vi "Length_9.vi"() -> ()   [LabVIEW 2020]
uses:
  Support/Controls/Cmd_Mouse Popup.ctl
  Support/Controls/Clst_Initialize Input.ctl
  Support/Controls/Cmd_Var Data IO.ctl
  Variables/Global_Cal Info.vi
panel:
  out "Spec 2":string[][](table) caption="Spec"
  out "Measured 2":string[][](table) caption="참고데이터"
  in  "체눈 수":string="10"
  in  "단위":string(combo)
  in  "선재 지름":string
  in  "체눈 크기":string
  in  "Spec 변경":bool
  in  "Random":bool
  out "Spec":string[][](table) caption="Spec Default"
  out "제목":string
  out "에러 출력":errorcluster
  out "Condition":string[][](table) caption="2. 직선성 시험"
  in  "Measured":string[][](table) caption="측정결과"
  out "Load?":bool
  # "※ 참고데이터는 기준기 보정값 적용하지 않은 체눈크기 계산 후 값임."
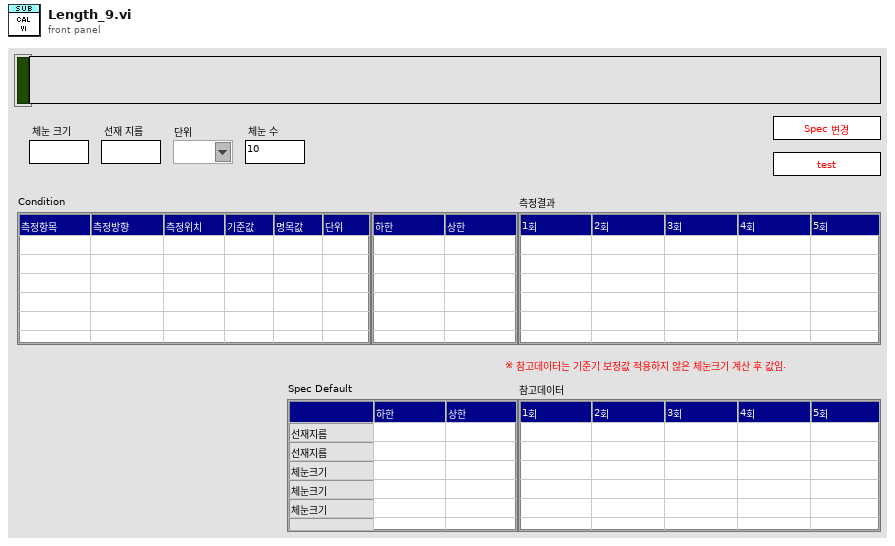
[diagram p1: front panel]
types:
  T1 = typedef "Cmd_Mouse Popup.ctl" = enum16{"활성화", "메뉴선택"}
  T2 = cluster{"Shift":bool, "Ctrl":bool, "Alt":bool, "Cmd":bool, "Opt":bool}
  T3 = typedef "Clst_Initialize Input.ctl" = cluster{"Initialize 1":cluster{"Condition":refnum<vi>[], "Spec":refnum<vi>[], "Measured":refnum<vi>[], "Resolution":refnum<vi>[], "Func_ext":string, "제목":refnum<vi>, "Measured_ADJ":refnum<vi>[]}, "Initialize 2":cluster{"문자열":refnum<vi>[], "콤보박스":refnum<vi>[], "링":refnum<vi>[], "열거형":refnum<vi>[], "테이블":refnum<vi>[], "여러열":refnum<vi>[], "디지털(DBL)":refnum<vi>[], "3D string":refnum<vi>[], "ctrl":refnum<vi>[], "boolean":refnum<vi>[]}}
  T4 = typedef "Cmd_Var Data IO.ctl" = enum16{"Condition", "Condition Default", "Condition_Temp", "Resolution", "Resolution Default", "Resolution Old", "Spec", "Spec Default", "Spec Old", "Spec Temp", "Result", "Result2", "Result3", "Result_Temp", "Result_ADJ", "Result_ADJ2", "STD1", "STD2", "STD3", "STD4", "STD5", "STD Temp", "CMC", "CMC Default"}
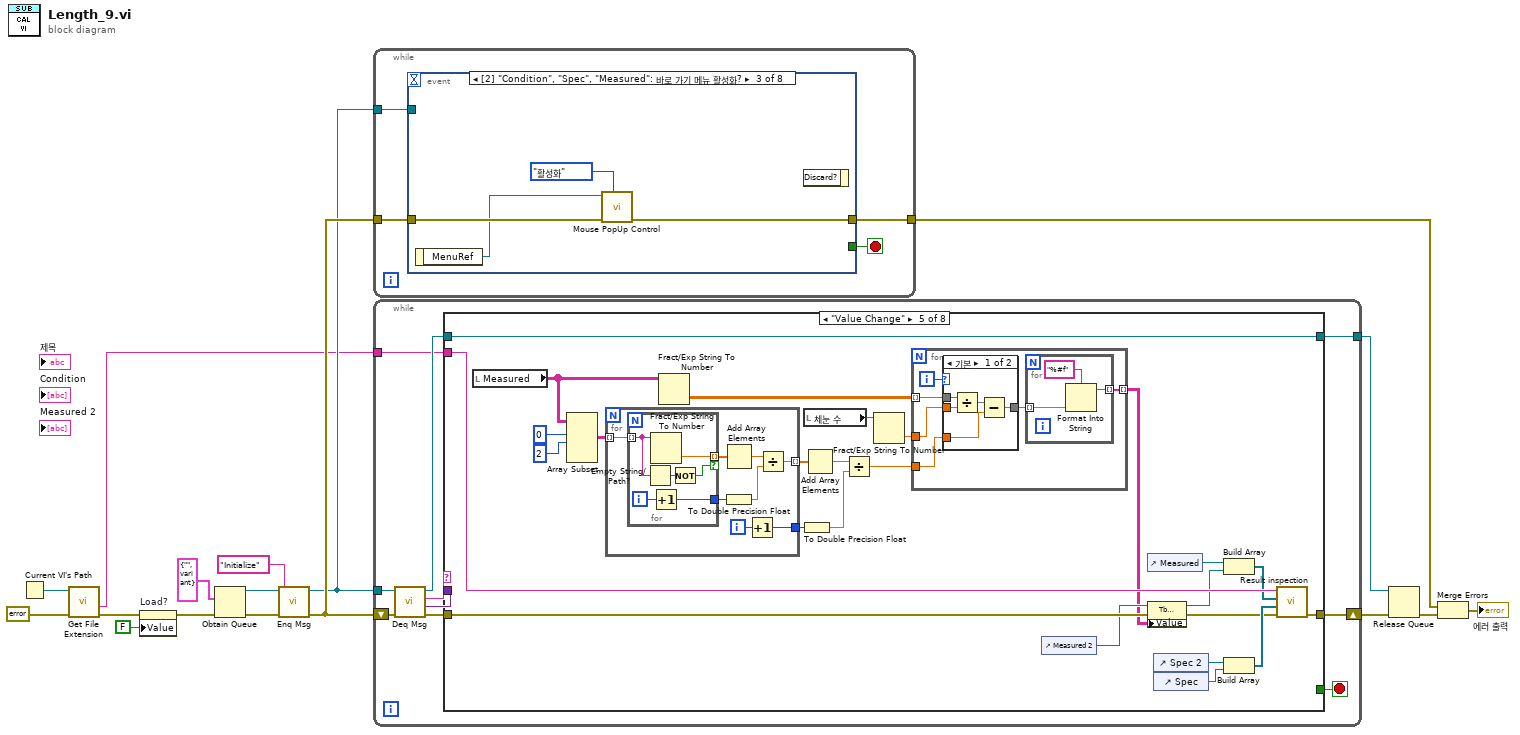
[diagram p0: block diagram]
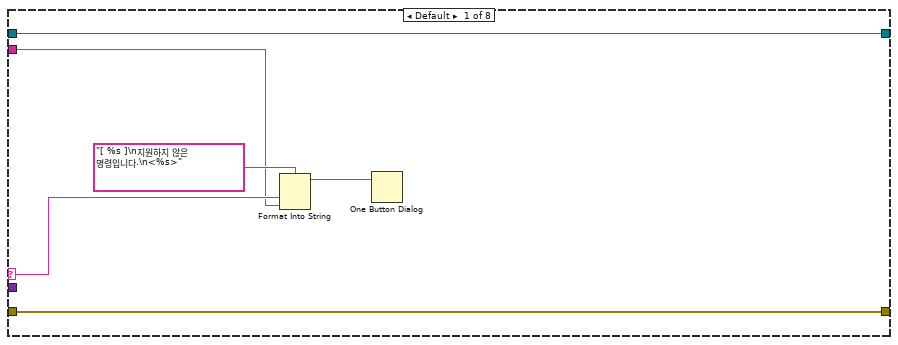
[diagram p2: hidden frame]
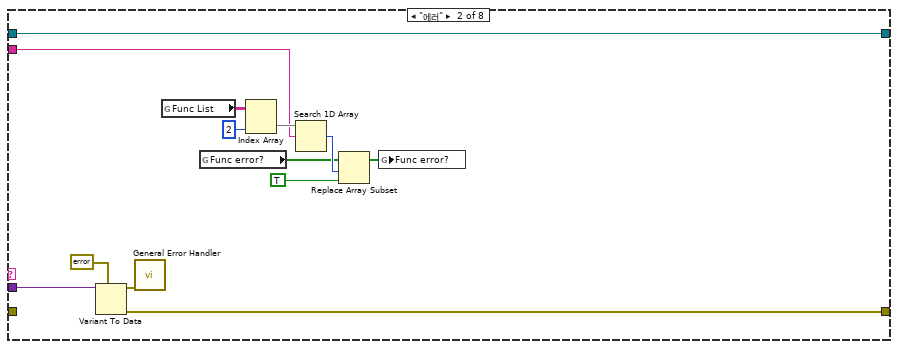
[diagram p3: hidden frame]
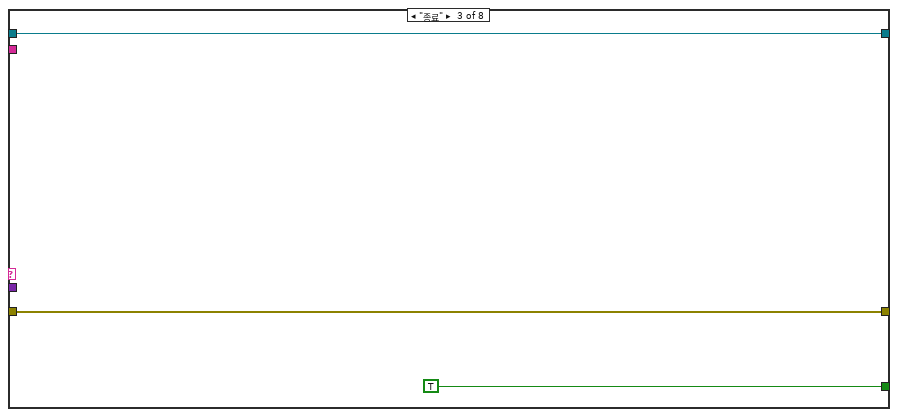
[diagram p4: hidden frame]
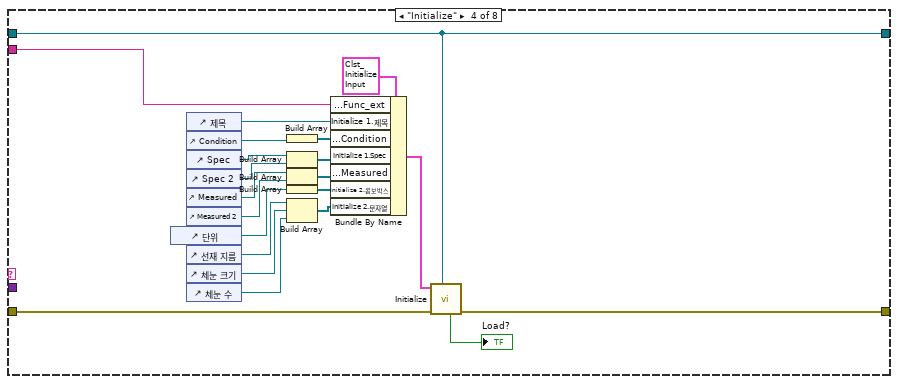
[diagram p5: hidden frame]
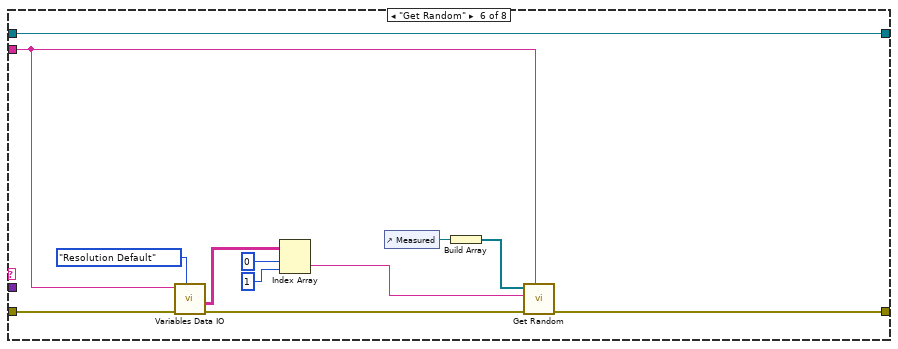
[diagram p7: hidden frame]
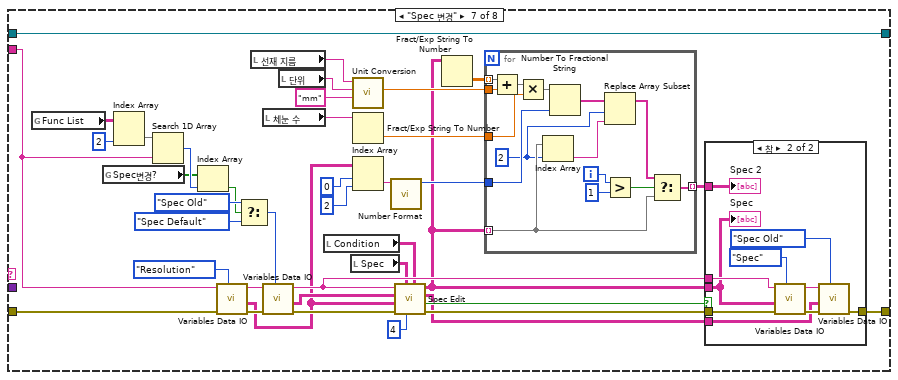
[diagram p8: hidden frame]
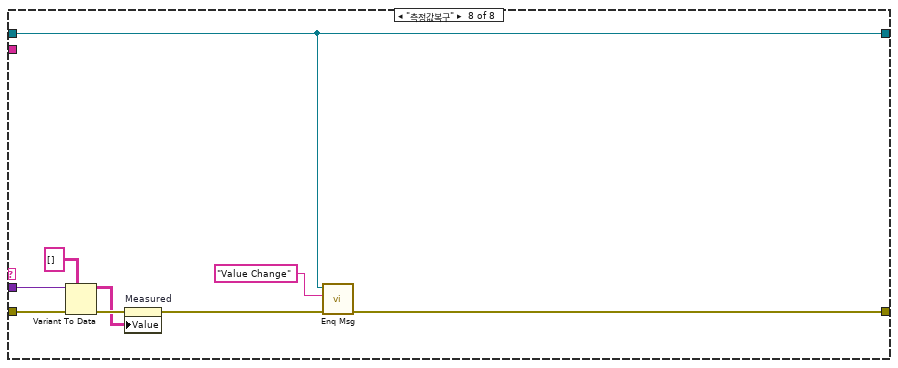
[diagram p10: hidden frame]
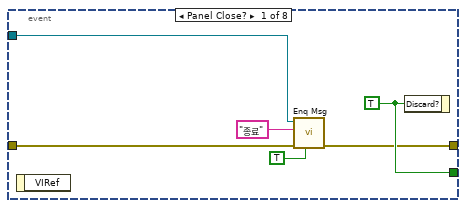
[diagram p11: hidden frame]
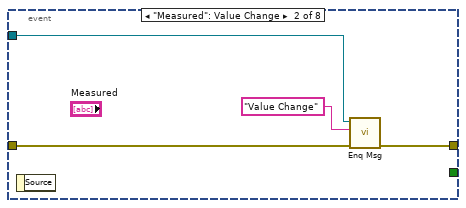
[diagram p12: hidden frame]
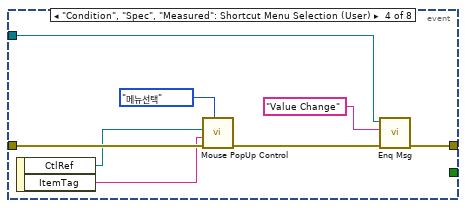
[diagram p13: hidden frame]
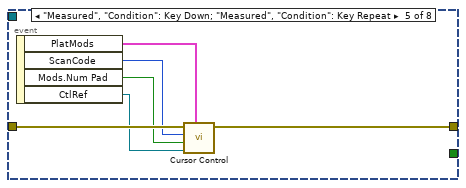
[diagram p14: hidden frame]
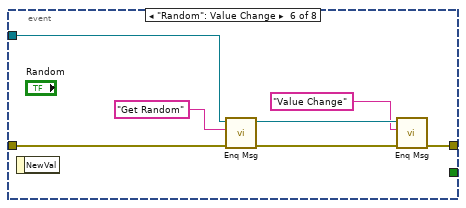
[diagram p15: hidden frame]
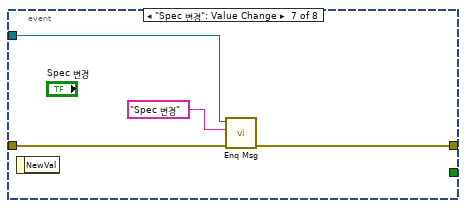
[diagram p16: hidden frame]
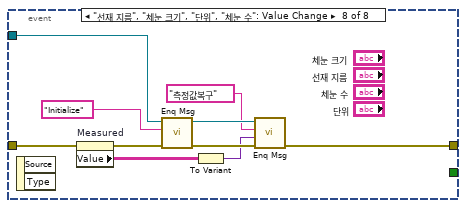
[diagram p17: hidden frame]
diagram:
  n1 = Current VI's Path() -> (path=w5:path)
  n2 = call <vilib>:"Get File Extension.vi"("error in (no error)"=errorcluster {"status"=FALSE, "code"=0, "source"=""} ("에러 상수"), "file"=w5) -> ("error out"=w3:errorcluster, "filename without extension"=w4:string)  [unwired: 5 in, 3 out]
  n3 = property on="Load?" class="Bool (엄격한)"(error in=w3, "Value"=FALSE ("Load?")) -> (error out=w2:errorcluster)  [unwired: 1 in, 1 out]
  n4 = Obtain Queue(element data type=cluster{"메세지":string, "값":variant} {"메세지"="", "값"=variant} ("Message Cluster"), error in (no error)=w2) -> (queue out=w14:refnum<queue>, error out=w16:errorcluster)  [unwired: 3 in, 1 out]
  n5 = call "Enq Msg.vi"("에러 입력(에러 없음)"=w16, "메세지"="Initialize", "큐 입력"=w14) -> ("에러 출력"=w15:errorcluster, "큐 출력"=w12:refnum<queue>)  [unwired: 7 in]
  n6 = while {
    tunnel: w15 -> [w19]
    tunnel: w12 -> [w20]
    tunnel: [w18] -> w9
    stop <- w21 stop-if-true
    n7 = event shown="[2] \"Condition\", \"Spec\", \"Measured\": 바로 가기 메뉴 활성화?" {
      selector: _ -> [_ _ _ _ _ _ _ _]
      dyn-events: _ -> [_ _ _ _ _ _ _ _]
      timeout: _ -> [_ _ _ _ _ _ _ _]
      tunnel: [w27 _ _ _ _ _ _ _] -> w21
      tunnel: w20 -> [w25 w31 _ w36 _ w54 w58 w69]
      tunnel: w19 -> [w26 w29 w35 w43 w49 w55 w59 w68]
      tunnel: [w23 w30 w34 w37 w48 w50 w57 w65] -> w18
      event Panel Close? {
        w27 = TRUE ("버림?")
        n8 = event-data() -> ()  [unwired: 1 in, 1 out]
        n9 = call "Enq Msg.vi"("우선순위 메시지?"=TRUE, "에러 입력(에러 없음)"=w26, "메세지"="종료", "큐 입력"=w25) -> ("에러 출력"=w23:errorcluster)  [unwired: 6 in, 1 out]
        n10 = event-data("Discard?"=w27) -> ()  [unwired: 1 in, 1 out]
      }
      event "Measured": Value Change {
        n11 = event-data() -> ()  [unwired: 1 in, 1 out]
        n12 = call "Enq Msg.vi"("에러 입력(에러 없음)"=w29, "메세지"="Value Change", "큐 입력"=w31) -> ("에러 출력"=w30:errorcluster)  [unwired: 7 in, 1 out]
      }
      event "Condition", "Spec", "Measured": Shortcut Menu Activation? {
        n13 = event-data() -> ("MenuRef"=w33:refnum<k9>)  [unwired: 1 in]
        n14 = call "Mouse PopUp Control.vi"("type"=Cmd_Mouse_Popup."활성화", "error in"=w35, "메뉴 참조"=w33) -> ("error out"=w34:errorcluster)  [unwired: 8 in]
        n15 = event-data() -> ()  [unwired: 2 in, 1 out]
      }
      event "Condition", "Spec", "Measured": Shortcut Menu Selection (User) {
        n16 = event-data() -> ("CtlRef"=w41:refnum<vi>, "ItemTag"=w40:string)  [unwired: 1 in]
        n17 = call "Mouse PopUp Control.vi"("type"=Cmd_Mouse_Popup."메뉴선택", "error in"=w43, "아이템 태그"=w40, "Tbl 참조 번호"=w41) -> ("error out"=w38:errorcluster)  [unwired: 7 in]
        n18 = call "Enq Msg.vi"("에러 입력(에러 없음)"=w38, "메세지"="Value Change", "큐 입력"=w36) -> ("에러 출력"=w37:errorcluster)  [unwired: 7 in, 1 out]
      }
      event "Measured", "Condition": Key Down; "Measured", "Condition": Key Repeat {
        n19 = event-data() -> ("PlatMods"=w44:T2, "ScanCode"=w47:i16, "Mods.Num Pad"=w46:bool, "CtlRef"=w45:refnum<vi>)  [unwired: 1 in]
        n20 = call "Cursor Control.vi"("플랫폼 조합키"=w44, "참조"=w45, "Num Pad"=w46, "ScanCode"=w47, "error in"=w49) -> ("error out"=w48:errorcluster)  [unwired: 5 in, 1 out]
      }
      event "Random": Value Change {
        n21 = event-data() -> ()  [unwired: 1 in, 1 out]
        n22 = call "Enq Msg.vi"("에러 입력(에러 없음)"=w55, "메세지"="Get Random", "큐 입력"=w54) -> ("에러 출력"=w53:errorcluster, "큐 출력"=w52:refnum<queue>)  [unwired: 7 in]
        n23 = call "Enq Msg.vi"("에러 입력(에러 없음)"=w53, "메세지"="Value Change", "큐 입력"=w52) -> ("에러 출력"=w50:errorcluster)  [unwired: 7 in, 1 out]
      }
      event "Spec 변경": Value Change {
        n24 = event-data() -> ()  [unwired: 1 in, 1 out]
        n25 = call "Enq Msg.vi"("에러 입력(에러 없음)"=w59, "메세지"="Spec 변경", "큐 입력"=w58) -> ("에러 출력"=w57:errorcluster)  [unwired: 7 in, 1 out]
      }
      event "선재 지름", "체눈 크기", "단위", "체눈 수": Value Change {
        n26 = event-data() -> ()  [unwired: 1 in, 2 out]
        n27 = property on="Measured" class="Tbl (엄격한)"(error in=w68) -> (error out=w67:errorcluster, "Value"=w61:string[][])  [unwired: 1 in, 1 out]
        n28 = call "Enq Msg.vi"("에러 입력(에러 없음)"=w67, "메세지"="Initialize", "큐 입력"=w69) -> ("에러 출력"=w66:errorcluster, "큐 출력"=w64:refnum<queue>)  [unwired: 7 in]
        n29 = To Variant(anything=w61) -> (Variant=w62:variant)
        n30 = call "Enq Msg.vi"("에러 입력(에러 없음)"=w66, "값"=w62, "메세지"="측정값복구", "큐 입력"=w64) -> ("에러 출력"=w65:errorcluster)  [unwired: 6 in, 1 out]
      }
    }
  }
  n31 = while {
    shift-right: [w80] -> w11
    shift-left: w15 -> [w79]
    tunnel: w12 -> [w77]
    tunnel: [w72] -> w10
    tunnel: w4 -> [w71]
    stop <- w73 stop-if-true
    n32 = call "Deq Msg.vi"("에러 입력(에러 없음)"=w79, "큐 입력"=w77) -> ("에러 출력"=w78:errorcluster, "값"=w74:variant, "메세지"=w76:string, "큐 출력"=w75:refnum<queue>)  [unwired: 6 in]
    n33 = case shown="\"Value Change\"" w76 {
      selector: w76 -> [w82 _ _ _ _ _ _ _]
      tunnel: w78 -> [w86 _ w102 w110 w137 w186 w209 w264]
      tunnel: [w86 w96 w102 w106 w148 w187 w226 w257] -> w80
      tunnel: w75 -> [w85 w95 w100 w114 w149 w190 w229 w256]
      tunnel: w74 -> [_ w97 _ _ _ _ _ w263]
      tunnel: [_ _ TRUE ("버림?") _ _ _ _ _] -> w73
      tunnel: [w85 w95 w100 w114 w149 w190 w229 w256] -> w72
      tunnel: w71 -> [w81 w87 _ w107 w147 w183 w207 _]
      frame Default {
        n34 = Format Into String(format string="[ %s ]\n지원하지 않은 명령입니다.\n<%s>" ("메시지"), w82, w81) -> (resulting string=w83:string)  [unwired: 2 in, 1 out]
        n35 = One Button Dialog(message=w83) -> ()  [unwired: 1 in, 1 out]
      }
      frame "에러" {
        n36 = Variant To Data(type=errorcluster {"status"=FALSE, "code"=0, "source"=""} ("에러 출력"), Variant=w97) -> (data=w99:errorcluster, error out=w96:errorcluster)  [unwired: 1 in]
        n37 = call <vilib>:"General Error Handler.vi"("error in (no error)"=w99) -> ()  [unwired: 10 in, 5 out]
        n38 = global read "Global_Cal Info.vi" "Func List"() -> (w89:string[][])
        n39 = global read "Global_Cal Info.vi" "Func error?"() -> (w92:bool[])
        n40 = Index Array(array=w89, index (col)=2 ("비활성화된 인덱스 (열)")) -> (element=w90:string[])  [unwired: 1 in]
        n41 = Search 1D Array(1D array=w90, element=w87) -> (index of element=w93:i32)  [unwired: 1 in]
        n42 = Replace Array Subset(array=w92, new element=TRUE ("새 원소/부분배열"), index=w93) -> (w94:bool[])
        n43 = global write "Global_Cal Info.vi" "Func error?"(w94) -> ()
      }
      frame "종료" {
      }
      frame "Initialize" {
        n44 = control-ref of="단위"() -> (w109:refnum<vi>)
        n45 = control-ref of="제목"() -> (w117:refnum<vi>)
        n46 = control-ref of="Condition"() -> (w122:refnum<vi>)
        n47 = control-ref of="Spec"() -> (w116:refnum<vi>)
        n48 = control-ref of="Spec 2"() -> (w105:refnum<vi>)
        n49 = control-ref of="Measured"() -> (w119:refnum<vi>)
        n50 = control-ref of="Measured 2"() -> (w104:refnum<vi>)
        n51 = control-ref of="선재 지름"() -> (w111:refnum<vi>)
        n52 = control-ref of="체눈 크기"() -> (w112:refnum<vi>)
        n53 = control-ref of="체눈 수"() -> (w108:refnum<vi>)
        n54 = Build Array(w122) -> (w121:refnum<vi>[])
        n55 = Build Array(w116, w105) -> (w115:refnum<vi>[])
        n56 = Build Array(w119, w104) -> (w120:refnum<vi>[])
        n57 = Build Array(w109) -> (w118:refnum<vi>[])
        n58 = Build Array(w111, w112, w108) -> (w113:refnum<vi>[])
        n59 = Bundle By Name(cluster=T3 {"Initialize 1"={"Condition"=[], "Spec"=[], "Measured"=[], "Resolution"=[], "Func_ext"="", "제목"=refnum, "Measured_ADJ"=[]}, "Initialize 2"={"문자열"=[], "콤보박스"=[], "링"=[], "열거형"=[], "테이블"=[], "여러열"=[], "디지털(DBL)"=[], "3D string"=[], "ctrl"=[], "boolean"=[]}} ("입력 클러스터"), "Initialize 1.Func_ext"=w107, "Initialize 1.제목"=w117, "Initialize 1.Condition"=w121, "Initialize 1.Spec"=w115, "Initialize 1.Measured"=w120, "Initialize 2.콤보박스"=w118, "Initialize 2.문자열"=w113) -> (w123:T3)
        n60 = call "Initialize.vi"("큐 입력"=w114, "error in"=w110, "입력 클러스터"=w123) -> ("error out"=w106:errorcluster, "Load?"=→"Load?":bool)  [unwired: 5 in, 2 out]
      }
      frame "Value Change" {
        n61 = local read "Measured"() -> (w130:string[][])
        n62 = Array Subset(array=w130, index (row)=0 ("인덱스"), length (row)=2 ("길이")) -> (w138:string[][])  [unwired: 2 in]
        n63 = for {
          tunnel: w138 -> [w155] mode=indexing
          tunnel: [w156] -> w129 mode=indexing
          tunnel: [w150] -> w128
          i -> [w151]
          n64 = for {
            tunnel: w155 -> [w163] mode=indexing
            tunnel: [w162] -> w154 mode=indexing if=w160
            tunnel: [w158] -> w153
            i -> [w159]
            n65 = Empty String/Path?(string/path=w163) -> (empty?=w161:bool)
            n66 = Fract/Exp String To Number(string=w163) -> (number=w162:dbl)  [unwired: 3 in, 1 out]
            n67 = Increment(x=w159) -> (x+1=w158:i32)
            n68 = Not(x=w161) -> (.not. x?=w160:bool)
          }
          n69 = Add Array Elements(numeric array=w154) -> (sum=w157:dbl)
          n70 = To Double Precision Float(number=w153) -> (double precision float=w152:dbl)
          n71 = Increment(x=w151) -> (x+1=w150:i32)
          n72 = Divide(x=w157, y=w152) -> (x/y=w156:dbl)
        }
        n73 = Fract/Exp String To Number(string=w130) -> (number=w141:dbl[][])  [unwired: 3 in, 1 out]
        n74 = To Double Precision Float(number=w128) -> (double precision float=w126:dbl)
        n75 = local read "체눈 수"() -> (w132:string)
        n76 = Add Array Elements(numeric array=w129) -> (sum=w127:dbl)
        n77 = Divide(x=w127, y=w126) -> (x/y=w125:dbl)
        n78 = Fract/Exp String To Number(string=w132) -> (number=w131:dbl)  [unwired: 3 in, 1 out]
        n79 = for {
          tunnel: w141 -> [w168] mode=indexing
          tunnel: w125 -> [w167]
          tunnel: [w165] -> w133 mode=indexing
          tunnel: w131 -> [w164]
          i -> [w169]
          n80 = case shown="기본" w169 {
            tunnel: w168 -> [w175 w178]
            tunnel: [w174 w178] -> w166
            tunnel: w167 -> [w173 _]
            tunnel: w164 -> [w176 _]
            frame Default {
              n81 = Divide(x=w175, y=w176) -> (x/y=w177:dbl[])
              n82 = Subtract(x=w177, y=w173) -> (x-y=w174:dbl[])
            }
            frame 0, 1 {
            }
          }
          n83 = for {
            tunnel: w166 -> [w172] mode=indexing
            tunnel: [w170] -> w165 mode=indexing
            n84 = Format Into String(format string="%#f" ("포맷 문자열"), w172) -> (resulting string=w170:string)  [unwired: 2 in, 1 out]
          }
        }
        n85 = control-ref of="Measured 2"() -> (w135:refnum<vi>)
        n86 = control-ref of="Measured"() -> (w146:refnum<vi>)
        n87 = property on="프로퍼티 노드" class="Tbl (엄격한)"(reference=w135, error in=w137, "Value"=w133) -> (reference out=w134:refnum<vi>, error out=w136:errorcluster)
        n88 = control-ref of="Spec 2"() -> (w144:refnum<vi>)
        n89 = control-ref of="Spec"() -> (w143:refnum<vi>)
        n90 = Build Array(w146, w134) -> (w145:refnum<vi>[])
        n91 = Build Array(w144, w143) -> (w142:refnum<vi>[])
        n92 = call "Result inspection.vi"("error in"=w136, "Ref. Data (excluded)"=w142, "Ref. Data (Inspection)"=w145, "Func ext"=w147) -> ("error out"=w148:errorcluster)  [unwired: 4 in, 3 out]
      }
      frame "Get Random" {
        n93 = call "Variables Data IO.vi"("Select"=Cmd_Var_Data_IO."Resolution Default", "error in"=w186, "Func_ext"=w183) -> ("error out"=w185:errorcluster, "Data Out"=w182:string[][])  [unwired: 6 in, 1 out]
        n94 = Index Array(array=w182, index (row)=0 ("인덱스 (행)"), index (col)=1 ("비활성화된 인덱스 (열)")) -> (element=w179:string)
        n95 = control-ref of="Measured"() -> (w189:refnum<vi>)
        n96 = Build Array(w189) -> (w188:refnum<vi>[])
        n97 = call "Get Random.vi"("Func_Ext"=w183, "에러 입력"=w185, "분해능"=w179, "Meas"=w188) -> ("에러 출력"=w187:errorcluster)  [unwired: 6 in, 1 out]
      }
      frame "Spec 변경" {
        n98 = global read "Global_Cal Info.vi" "Func List"() -> (w216:string[][])
        n99 = global read "Global_Cal Info.vi" "Spec변경?"() -> (w212:bool[])
        n100 = Index Array(array=w216, index (col)=2 ("비활성화된 인덱스 (열)")) -> (element=w214:string[])  [unwired: 1 in]
        n101 = Search 1D Array(1D array=w214, element=w207) -> (index of element=w213:i32)  [unwired: 1 in]
        n102 = Index Array(array=w212, index=w213) -> (element=w217:bool)
        n103 = call "Variables Data IO.vi"("Select"=Cmd_Var_Data_IO."Resolution", "error in"=w209, "Func_ext"=w207) -> ("error out"=w210:errorcluster, "Data Out"=w202:string[][], "Func_ext Out"=w208:string)  [unwired: 6 in]
        n104 = Select(t=Cmd_Var_Data_IO."Spec Old" ("Select"), s=w217, f=Cmd_Var_Data_IO."Spec Default" ("Select")) -> (s? t:f=w211:T4)
        n105 = local read "선재 지름"() -> (w194:string)
        n106 = local read "체눈 수"() -> (w198:string)
        n107 = call "Variables Data IO.vi"("Select"=w211, "error in"=w210, "Func_ext"=w208) -> ("error out"=w225:errorcluster, "Data Out"=w220:string[][], "Func_ext Out"=w221:string)  [unwired: 6 in]
        n108 = local read "단위"() -> (w193:string)
        n109 = local read "Condition"() -> (w206:string[][])
        n110 = local read "Spec"() -> (w199:string[][])
        n111 = call "Unit Conversion.vi"("환산단위"="mm" ("포맷 문자열"), "입력단위"=w193, "입력값"=w194) -> ("환산값 (DBL)"=w195:dbl)  [unwired: 3 in, 5 out]
        n112 = Fract/Exp String To Number(string=w198) -> (number=w197:dbl)  [unwired: 3 in, 1 out]
        n113 = Index Array(array=w202, index (row)=0 ("인덱스 (행)"), index (col)=2 ("비활성화된 인덱스 (열)")) -> (element=w203:string)
        n114 = call "Number Format.vi"("입력값"=w203) -> ("정밀도(단위적용)"=w204:i32)  [unwired: 10 in]
        n115 = call "Spec Edit.vi"("Condition"=w206, "열번호(기준값)"=4, "Spec Value"=w199, "에러 입력(에러 없음)"=w225, "Resolution"=w202, "Spec Default"=w220, "Func_ext"=w221) -> ("에러 출력"=w227:errorcluster, "변경?"=w228:bool, "Spec Default out"=w223:string[][], "Spec 출력"=w191:string[][])  [unwired: 1 in]
        n116 = Fract/Exp String To Number(string=w191) -> (number=w205:dbl[][])  [unwired: 3 in, 1 out]
        n117 = for {
          tunnel: w205 -> [w244] mode=indexing
          tunnel: w195 -> [w243]
          tunnel: w197 -> [w241]
          tunnel: [w231] -> w196 mode=indexing
          tunnel: w191 -> [w235] mode=indexing
          tunnel: w204 -> [w237]
          i -> [w234]
          w230 = 2 ("인덱스")
          n118 = Add(x=w244, y=w243) -> (x+y=w242:dbl[])
          n119 = Multiply(x=w242, y=w241) -> (x*y=w240:dbl[])
          n120 = Index Array(array=w235, index=w230) -> (element=w238:string)
          n121 = Number To Fractional String(number=w240, precision (6)=w237) -> (F-format string=w239:string[])  [unwired: 2 in]
          n122 = Replace Array Subset(array=w239, new element=w238, index=w230) -> (w236:string[])
          n123 = Greater?(x=w234, y=1) -> (0:w232:bool)
          n124 = Select(t=w236, s=w232, f=w235) -> (s? t:f=w231:string[])
        }
        n125 = case shown="참" w228 {
          tunnel: w191 -> [_ w252]
          tunnel: w227 -> [w245 w255]
          tunnel: [w245 w250] -> w226
          tunnel: w221 -> [_ w253]
          tunnel: w223 -> [_ w248]
          tunnel: w196 -> [_ w246]
          frame False {
          }
          frame True {
            n126 = call "Variables Data IO.vi"("Select"=Cmd_Var_Data_IO."Spec", "error in"=w255, "Data In"=w252, "Func_ext"=w253) -> ("error out"=w251:errorcluster, "Func_ext Out"=w249:string)  [unwired: 5 in, 1 out]
            n127 = call "Variables Data IO.vi"("Select"=Cmd_Var_Data_IO."Spec Old", "error in"=w251, "Data In"=w248, "Func_ext"=w249) -> ("error out"=w250:errorcluster)  [unwired: 5 in, 2 out]
            "Spec" <- w252
            "Spec 2" <- w246
          }
        }
      }
      frame "측정값복구" {
        n128 = Variant To Data(error in=w264, type=string[][] [], Variant=w263) -> (data=w260:string[][], error out=w261:errorcluster)
        n129 = property on="Measured" class="Tbl (엄격한)"(error in=w261, "Value"=w260) -> (error out=w258:errorcluster)  [unwired: 1 in, 1 out]
        n130 = call "Enq Msg.vi"("에러 입력(에러 없음)"=w258, "메세지"="Value Change", "큐 입력"=w256) -> ("에러 출력"=w257:errorcluster)  [unwired: 7 in, 1 out]
      }
    }
  }
  n131 = Release Queue(queue=w10, error in (no error)=w11) -> (error out=w8:errorcluster)  [unwired: 1 in, 2 out]
  n132 = Merge Errors(w9, w8) -> (→"에러 출력":errorcluster)
